vi "Color to RGB.vi"(4 "Color":u32(colorbox)) -> (1 "32bit out":u32)   [LabVIEW 2020, in "lvpptx.lvlib"]
uses:
  lvpptx.lvlib
panel:
  # "Converts LabVIEW color to int32\nthat represents color in MS Office"
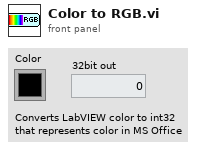
[diagram p1: front panel]
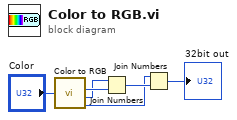
[diagram p0: block diagram]
diagram:
  n1 = call <vilib>:"Color to RGB.vi"("Color"="Color") -> ("R"=w6:u8, "G"=w5:u8, "B"=w3:u8)  [unwired: 1 out]
  n2 = Join Numbers(hi=w5, lo=w6) -> ((hi.lo)=w4:u16)
  n3 = Join Numbers(hi=w3, lo=w4) -> ((hi.lo)=→"32bit out":u32)
